vi "Init.vi"(1 "Results queue":refnum<queue>, 4 "Pre-preocess datasockets":bool, 5 "Caller Enqueuer":refnum<class "Message Enqueuer.lvclass">, 6 "Subscribe":bool, 7 "Self Enqueuer":refnum<class "Message Enqueuer.lvclass">, 8 "error in (no error)":errorcluster, 9 "Topics":string[](array[string])=["Result"], 10 "Responder names":string[](array[string]), 11 "Response Synchronizer in":refnum<class "Response Synchronizer.lvclass">) -> (0 "error out":errorcluster, 2 "Result ready":bool, 3 "Response Synchronizer out":refnum<class "Response Synchronizer.lvclass">)   [LabVIEW 2024, in "Response Synchronizer.lvclass"]
uses:
  Response Synchronizer.lvclass
  <vilib>/ActorFramework/Message Enqueuer/Message Enqueuer.lvclass
  NHMFL_Core/Libraries/Instruments/Results/Acquired Result/Acquired Result.lvclass
  Response Synchronizer.lvclass/Response Synchronizer.ctl
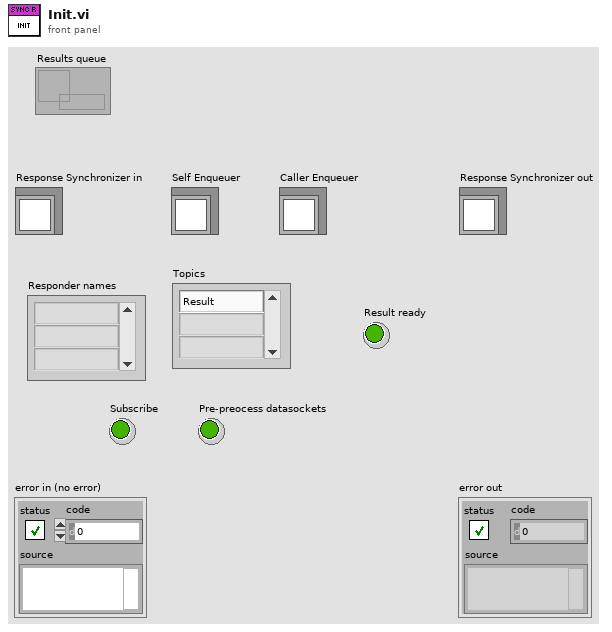
[diagram p1: front panel]
types:
  T1 = map{cluster{"Accessors:Sender":string, "Accessors:Cycle count":i32}, refnum<class "Acquired Result.lvclass">}
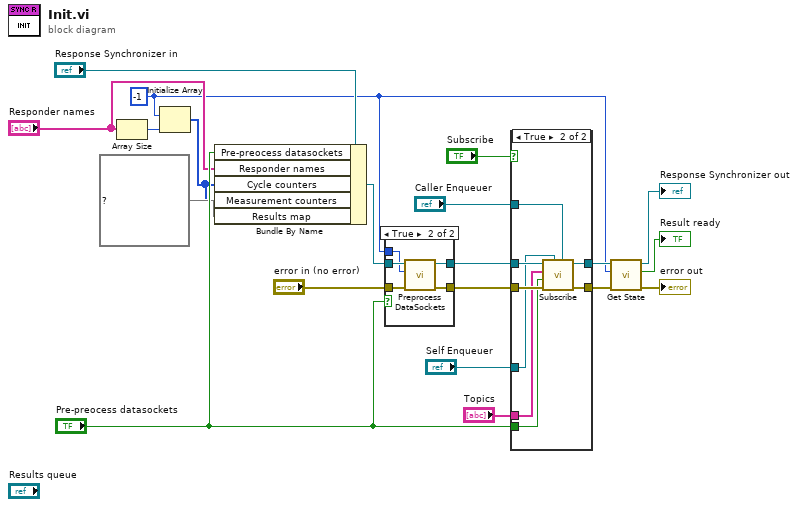
[diagram p0: block diagram]
diagram:
  w2 = -1 ("Numeric")
  n1 = Array Size(array="Responder names") -> (size(s)=w4:i32)
  n2 = Initialize Array(w2, w4) -> (w1:i32[])
  n3 = Bundle By Name(cluster="Response Synchronizer in", "Pre-preocess datasockets"="Pre-preocess datasockets", "Responder names"="Responder names", "Cycle counters"=w1, "Measurement counters"=w1, "Results map"=T1 {}) -> (w11:refnum<class "Response Synchronizer.lvclass">)
  n4 = case shown="True" "Pre-preocess datasockets" {
    tunnel: "error in (no error)" -> [w21 w27]
    tunnel: [w21 w26] -> w9
    tunnel: w11 -> [w22 w25]
    tunnel: [w22 w24] -> w8
    tunnel: w2 -> [_ w23]
    frame False {
    }
    frame True {
      n5 = call-dynamic "Preprocess DataSockets.vi"("error in (no error)"=w27, "Cycle count"=w23, "Response Synchronizer in"=w25) -> ("error out"=w26:errorcluster, "Response Synchronizer out"=w24:refnum<class "Response Synchronizer.lvclass">)  [unwired: 7 in]
    }
  }
  n6 = case shown="True" "Subscribe" {
    tunnel: w9 -> [w29 w36]
    tunnel: "Caller Enqueuer" -> [_ w37]
    tunnel: w8 -> [w28 w35]
    tunnel: [w28 w34] -> w17
    tunnel: [w29 w33] -> w16
    tunnel: "Self Enqueuer" -> [_ w32]
    tunnel: "Pre-preocess datasockets" -> [_ w31]
    tunnel: "Topics" -> [_ w30]
    frame False {
    }
    frame True {
      n7 = call-dynamic "Subscribe.vi"("Caller Enqueuer"=w37, "Self Enqueuer"=w32, "error in (no error)"=w36, "Pre-preocess datasockets"=w31, "Topics"=w30, "Response Synchronizer in"=w35) -> ("error out"=w33:errorcluster, "Response Synchronizer out"=w34:refnum<class "Response Synchronizer.lvclass">)  [unwired: 4 in]
    }
  }
  n8 = call-dynamic "Get State.vi"("error in (no error)"=w16, "Cycle count"=w2, "Response Synchronizer in"=w17) -> ("error out"=→"error out":errorcluster, "Result ready"=→"Result ready":bool, "Response Synchronizer out"=→"Response Synchronizer out":refnum<class "Response Synchronizer.lvclass">)  [unwired: 2 in, 4 out]
